vi "modify channel test.vi"() -> (0 "no err":errorcluster, 3 "mod success":bool)   [LabVIEW 2015, in "PID Module tests.lvlib"]
doc: "Tests the 'Replace Line' VI."
uses:
  PID Module tests.lvlib
  <vilib>/NI/Tag Bus Module Framework/channel/TBM channel.lvclass/TBM channel.ctl
  <vilib>/NI/Tag Bus Module Framework/channel/channel classification.ctl
  <vilib>/NI/Tag Bus/tag/tag descriptor.lvclass/tag descriptor.ctl
  <vilib>/NI/Tag Bus Module Framework/channel/Read channel classification.vi
  <vilib>/NI/Tag Bus Module Framework/channel/Write channel classification.vi
  <vilib>/NI/Tag Bus/tag/read tag name.vi
  module/configuration/PID Module configuration.lvclass
  <vilib>/NI/Tag Bus Module Framework/channel/TBM channel.lvclass
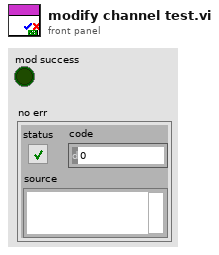
[diagram p1: front panel]
types:
  T1 = typedef "PID Module configuration.lvclass/Line.ctl" = cluster{"PID ID":string, "Setpoint":refnum<class "TBM channel.lvclass">, "Variable":refnum<class "TBM channel.lvclass">, "Output":refnum<class "TBM channel.lvclass">, "Output High":refnum<class "TBM channel.lvclass">, "Output Low":refnum<class "TBM channel.lvclass">, "P":refnum<class "TBM channel.lvclass">, "I":refnum<class "TBM channel.lvclass">, "D":refnum<class "TBM channel.lvclass">}
  T2 = typedef "TBM channel.lvclass/channel classification.ctl" = enum16{"input data", "output data", "processing parameter", "processing result"}
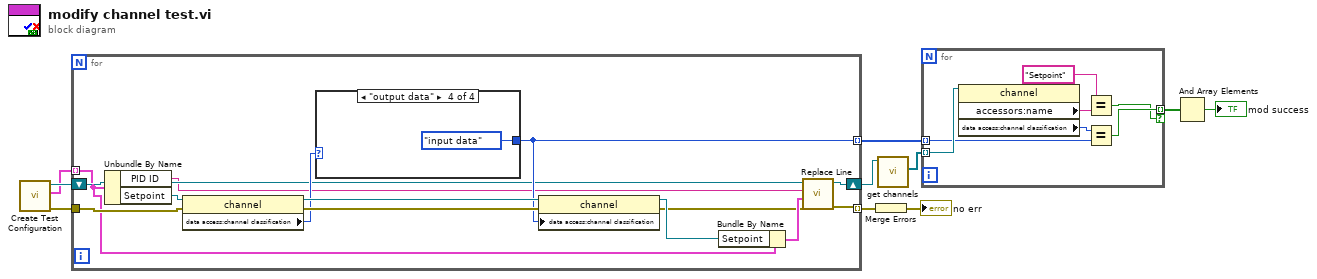
[diagram p0: block diagram]
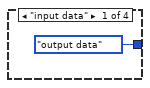
[diagram p2: hidden frame]
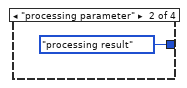
[diagram p3: hidden frame]
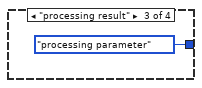
[diagram p4: hidden frame]
diagram:
  n1 = call "Create Test Configuration.vi"() -> ("error out"=w3:errorcluster, "Line Array"=w4:T1[], "Module Configuration"=w5:refnum<class "PID Module configuration.lvclass">)  [unwired: 6 in, 3 out]
  n2 = for {
    shift-right: [w17] -> w10
    shift-left: w5 -> [w16]
    tunnel: w4 -> [w15] mode=indexing
    tunnel: [w20] -> w6 mode=indexing
    tunnel: w3 -> [w24]
    tunnel: [w18] -> w9 mode=indexing
    n3 = Unbundle By Name(w15) -> ("PID ID"=w12:string, "Setpoint"=w19:refnum<class "TBM channel.lvclass">)
    n4 = property class="channel"(reference=w19, error in=w24) -> (reference out=w22:refnum<class "TBM channel.lvclass">, error out=w23:errorcluster, "data access:channel classification"=w21:T2)
    n5 = case shown="\"output data\"" w21 {
      tunnel: [channel_classification."output data" ("channel classification") channel_classification."processing result" ("channel classification") channel_classification."processing parameter" ("channel classification") channel_classification."input data" ("channel classification")] -> w20
      frame "input data" {
      }
      frame "processing parameter" {
      }
      frame "processing result" {
      }
      frame "output data" {
      }
    }
    n6 = property class="channel"(reference=w22, error in=w23, "data access:channel classification"=w20) -> (reference out=w13:refnum<class "TBM channel.lvclass">, error out=w11:errorcluster)
    n7 = Bundle By Name(cluster=w15, "Setpoint"=w13) -> (w14:T1)
    n8 = call "Replace Line.vi"("error in"=w11, "New Line"=w14, "Line Name"=w12, "PID Module 2 configuration in"=w16) -> ("error out"=w18:errorcluster, "PID Module 2 configuration out"=w17:refnum<class "PID Module configuration.lvclass">)  [unwired: 5 in, 1 out]
  }
  n9 = Merge Errors(w9) -> (→"no err":errorcluster)
  n10 = call-dynamic "get channels.vi"("PID Module 2 configuration in"=w10) -> ("channels"=w8:refnum<class "TBM channel.lvclass">[])  [unwired: 9 in, 1 out]
  n11 = for {
    tunnel: w8 -> [w35] mode=indexing
    tunnel: w6 -> [w34] mode=indexing
    tunnel: [w30] -> w1 mode=indexing if=w29
    n12 = property class="channel"(reference=w35) -> ("accessors:name"=w32:string, "data access:channel classification"=w33:T2)  [unwired: 1 in, 2 out]
    n13 = Equal?(x="Setpoint", y=w32) -> (x = y?=w29:bool)
    n14 = Equal?(x=w33, y=w34) -> (x = y?=w30:bool)
  }
  n15 = And Array Elements(Boolean array=w1) -> (logical AND=→"mod success":bool)
